vi "Main_Transfer_LaunchPy.vi"() -> ()   [LabVIEW 2020]
uses:
  <vilib>/vision/NI_Vision_Development_Module.lvlib
panel:
  in  "h":i32=10 min=1 max=5000 step=1
  in  "w":i32=1 min=1 max=5000 step=1
  out "Elaps ms":u32
  in  "Send Image":bool
  out "Path to Python script":path
  in  "Stop":bool
  out "Answer":string
  in  "Ping":bool
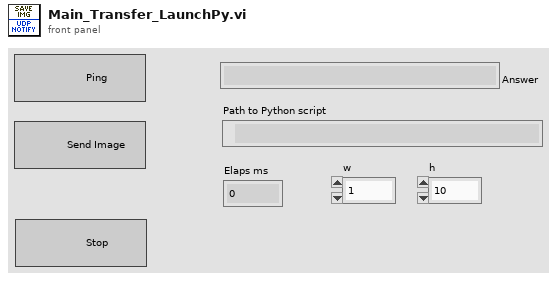
[diagram p1: front panel]
types:
  T1 = enum8{"Enabled", "Disabled", "Disabled and Grayed Out"}
  T2 = typedef "Image Type" = u32
  T3 = cluster{"Rows Per Strip":i32, "Photometric":i32, "Compression Type":i32}
  T4 = typedef "IMAQ Image.ctl" = refnum<image>
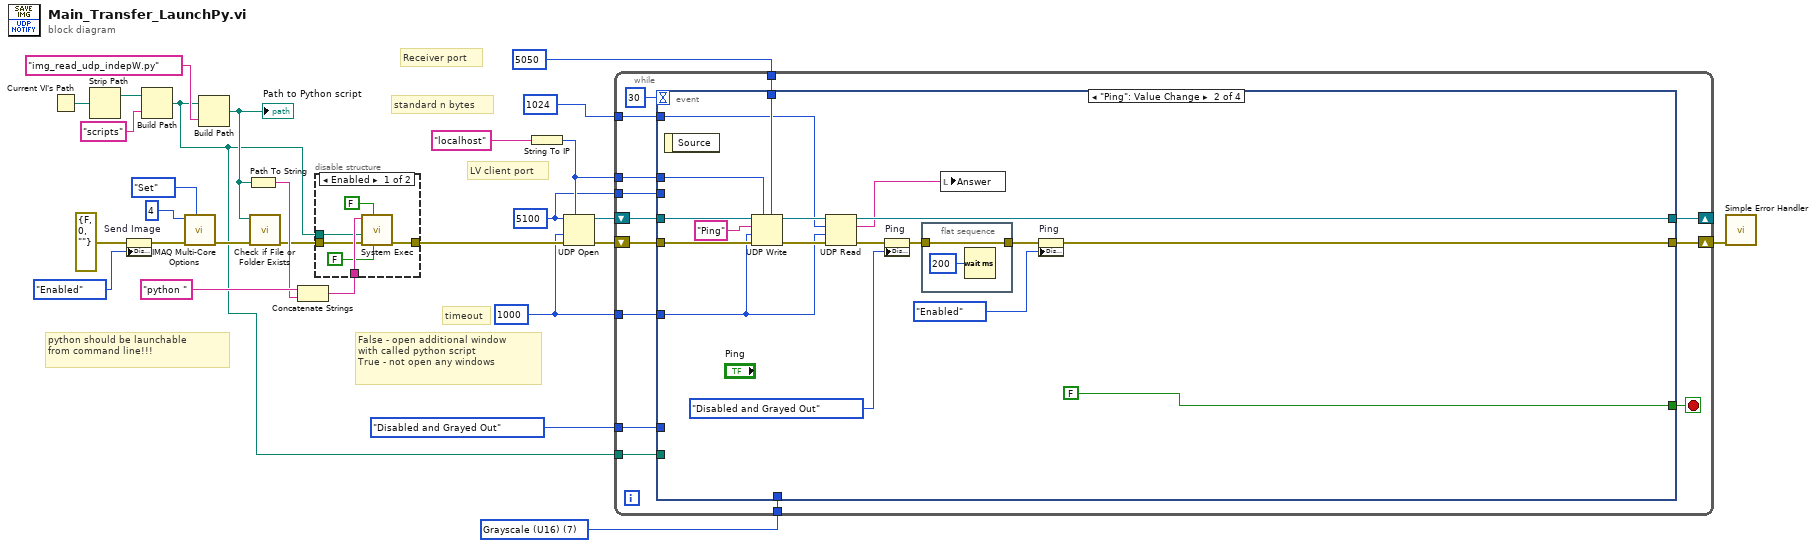
[diagram p0: block diagram]
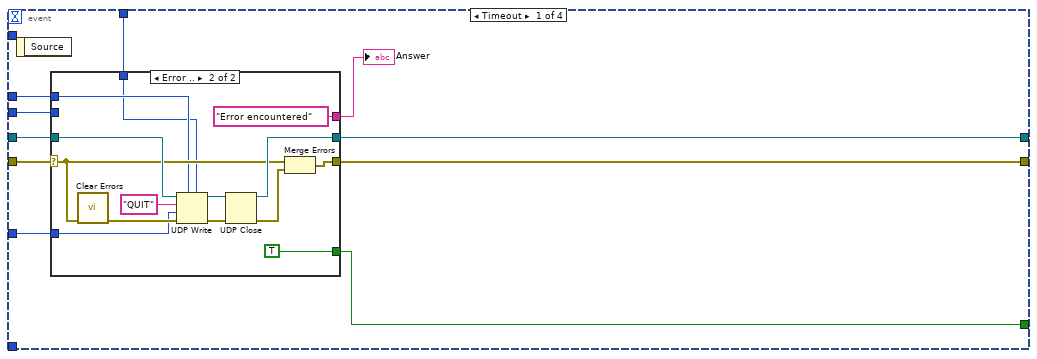
[diagram p3: hidden frame]
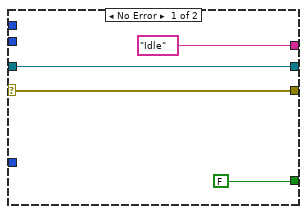
[diagram p4: hidden frame]
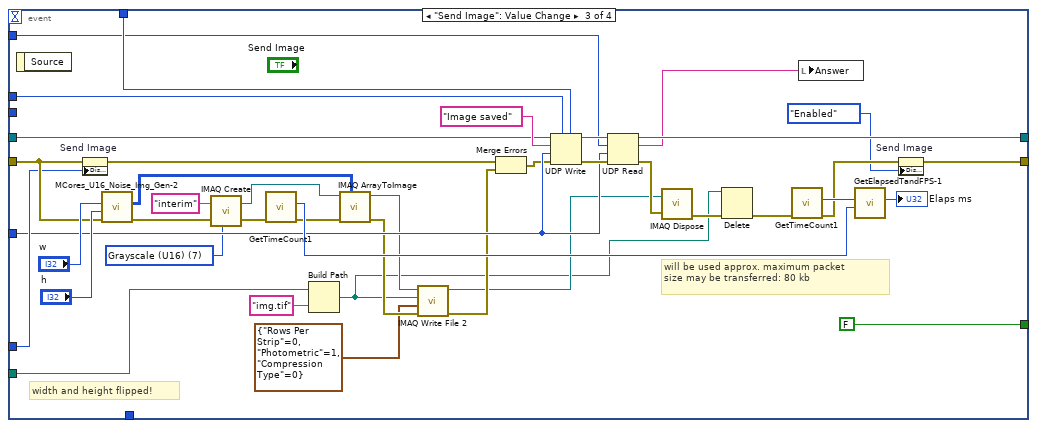
[diagram p5: hidden frame]
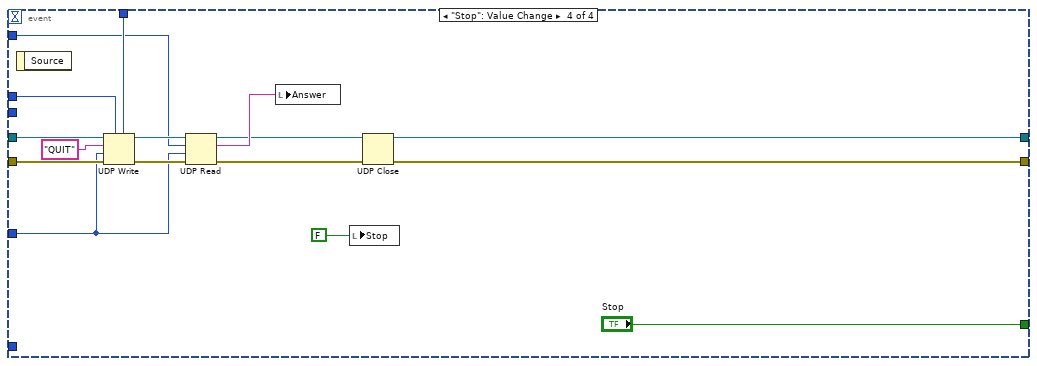
[diagram p6: hidden frame]
diagram:
  w13 = T2 7 items=["Grayscale (U8)", "Grayscale (I16)", "Grayscale (SGL)", "Complex (CSG)", "RGB (U32)", "HSL (U32)", "RGB (U64)", "Grayscale (U16)"] ("Image Type")
  w1 = 1000
  w15 = u16 5100 ("remote port or service name")
  # "standard n bytes"
  # "timeout"
  # "Receiver port"
  # "LV client port"
  # "False - open additional window\nwith called python script\nTrue - not open any windows"
  # "python should be launchable \nfrom command line!!!"
  n1 = Current VI's Path() -> (path=w27:path)
  n2 = Strip Path(path=w27) -> (stripped path=w3:path)  [unwired: 1 out]
  n3 = property on="Send Image" class="Bool"(error in=errorcluster {"status"=FALSE, "code"=0, "source"=""} ("error in (no error)"), "DisabledEnum"=T1."Enabled" ("Disabled")) -> (error out=w7:errorcluster)  [unwired: 1 in, 1 out]
  n4 = Build Path(base path=w3, name or relative path="scripts" ("string")) -> (appended path=w2:path)
  n5 = call "IMAQ Multi-Core Options"("Get/Set Number of Cores (Get)"=enum32{"Get", "Set", "Set Max Available"}."Set", "error in (no error)"=w7, "Specified Number of Cores"=u32 4) -> ("error out"=w4:errorcluster)  [unwired: 7 in, 1 out]
  n6 = Build Path(base path=w2, name or relative path="img_read_udp_indepW.py" ("string")) -> (appended path=w22:path)
  "Path to Python script" <- w22
  n7 = Path To String(path=w22) -> (string=w23:string)
  n8 = call <vilib>:"Check if File or Folder Exists.vi"("error in (no error)"=w4, "path"=w22) -> ("error out"=w21:errorcluster)  [unwired: 7 in, 2 out]
  n9 = Concatenate Strings("python " ("command line"), w23) -> (w25:string)
  n10 = disable-structure shown="Enabled" {
    disable-tunnel: w25 -> [w34 _]
    disable-tunnel: [w33 w35] -> w20
    disable-tunnel: w21 -> [w31 w35]
    disable-tunnel: w2 -> [w29 _]
    frame Enabled {
      n11 = call <vilib>:"System Exec.vi"("run minimized? (F)"=FALSE, "wait until completion? (T)"=FALSE, "error in (no error)"=w31, "working directory"=w29, "command line"=w34) -> ("error out"=w33:errorcluster)  [unwired: 3 in, 3 out]
    }
    frame Disabled {
    }
  }
  n12 = String To IP(1:"localhost" ("address")) -> (0:w16:u32)
  n13 = UDP Open(7:w16, 8:w20, 9:w1, 11:w15) -> (port=w18:refnum<k16>, 0:w19:errorcluster)  [unwired: 1 in, 1 out]
  n14 = while {
    shift-right: [w46] -> _
    shift-left: w18 -> [w47]
    shift-right: [w44] -> w28
    shift-left: w19 -> [w48]
    tunnel: w16 -> [w42]
    tunnel: w15 -> [w43]
    tunnel: u16 5050 ("remote port or service name") -> [w41]
    tunnel: w1 -> [w40]
    tunnel: w13 -> [w39]
    tunnel: T1."Disabled and Grayed Out" ("Disabled") -> [w38]
    tunnel: 1024 ("bytes to read") -> [w37]
    tunnel: w2 -> [w36]
    stop <- w45 stop-if-true
    n15 = event shown="[1] \"Ping\": Value Change" {
      selector: _ -> [_ _ _ _]
      dyn-events: _ -> [_ _ _ _]
      timeout: 30 -> [_ _ _ _]
      tunnel: [w55 FALSE ("Stop") FALSE ("Stop") "Stop"] -> w45
      tunnel: w48 -> [w59 w89 w126 w149]
      tunnel: w47 -> [w58 w88 w137 w150]
      tunnel: [w57 w84 w135 w151] -> w46
      tunnel: [w56 w91 w123 w152] -> w44
      tunnel: w43 -> [w53 _ _ _]
      tunnel: w42 -> [w52 w81 w130 w142]
      tunnel: w41 -> [w51 w80 w129 w141]
      tunnel: w40 -> [w50 w79 w119 w139]
      tunnel: w39 -> [_ _ _ _]
      tunnel: w38 -> [_ _ w125 _]
      tunnel: w37 -> [_ w78 w118 w140]
      tunnel: w36 -> [_ _ w104 _]
      event Timeout {
        n16 = event-data() -> ()  [unwired: 1 in, 1 out]
        n17 = case shown="Error .." w59 {
          selector: w59 -> [w62 w68]
          tunnel: [w63 w75] -> w57
          tunnel: w58 -> [w63 w74]
          tunnel: [w62 w69] -> w56
          tunnel: [FALSE ("Stop") TRUE ("Stop")] -> w55
          tunnel: ["Idle" ("Answer") "Error encountered" ("Answer")] -> w54
          tunnel: w53 -> [_ _]
          tunnel: w52 -> [_ w66]
          tunnel: w51 -> [_ w65]
          tunnel: w50 -> [_ w64]
          frame No Error {
          }
          frame Error {
            n18 = call <vilib>:"Clear Errors.vi"("error in (no error)"=w68) -> ("error out"=w73:errorcluster)  [unwired: 5 in, 1 out]
            n19 = UDP Write(address=w66, port or service name=w65, connection ID=w74, data in="QUIT", 8:w73, 9:w64) -> (error out=w72:errorcluster, 3:w70:refnum<k16>)
            n20 = UDP Close(connection ID=w70, 8:w72) -> (connection ID out=w75:refnum<k16>, error out=w67:errorcluster)
            n21 = Merge Errors(w68, w67) -> (w69:errorcluster)
          }
        }
        "Answer" <- w54
      }
      event "Ping": Value Change {
        n22 = event-data() -> ()  [unwired: 1 in, 1 out]
        n23 = UDP Write(address=w81, port or service name=w80, connection ID=w88, data in="Ping", 8:w89, 9:w79) -> (error out=w86:errorcluster, 3:w85:refnum<k16>)
        n24 = UDP Read(connection ID=w85, max size (548)=w78, timeout ms (25000)=w79, 8:w86) -> (data out=w82:string, error out=w83:errorcluster, 3:w84:refnum<k16>)  [unwired: 2 out]
        n25 = property on="Ping" class="Bool"(error in=w83, "DisabledEnum"=T1."Disabled and Grayed Out" ("Disabled")) -> (error out=w94:errorcluster)  [unwired: 1 in, 1 out]
        n26 = flat-sequence {
          tunnel: w94 -> [w96]
          tunnel: [w96] -> w92
          frame #0 {
            n27 = Wait (ms)(milliseconds to wait=u32 200) -> ()  [unwired: 1 out]
          }
        }
        n28 = local write "Answer"(w82) -> ()
        n29 = property on="Ping" class="Bool"(error in=w92, "DisabledEnum"=T1."Enabled" ("Disabled")) -> (error out=w91:errorcluster)  [unwired: 1 in, 1 out]
      }
      event "Send Image": Value Change {
        w115 = T2 7 items=["Grayscale (U8)", "Grayscale (I16)", "Grayscale (SGL)", "Complex (CSG)", "RGB (U32)", "HSL (U32)", "RGB (U64)", "Grayscale (U16)"] ("Image Type")
        # "width and height flipped!"
        # "will be used approx. maximum packet \nsize may be transferred: 80 kb"
        n30 = event-data() -> ()  [unwired: 1 in, 1 out]
        n31 = property on="Send Image" class="Bool"(error in=w126, "DisabledEnum"=w125) -> (error out=w117:errorcluster)  [unwired: 1 in, 1 out]
        n32 = call "MCores_U16_Noise_Img_Gen-2.vi"("error IN"=w126, "[IN] Width"="h", "[IN] Height"="w") -> ("error OUT"=w113:errorcluster, "[OUT] U16 Pixel Img"=w109:u16[][])  [unwired: 7 in]
        n33 = call "IMAQ Create"("Image Name"="interim", "Image Type"=w115, "error in (no error)"=w113) -> ("New Image"=w110:T4, "error out"=w112:errorcluster)  [unwired: 2 in]
        n34 = call "GetTimeCount1.vi"("error IN"=w112) -> ("error OUT"=w111:errorcluster, "[OUT] Timer Count"=w132:u32)  [unwired: 9 in]
        n35 = Build Path(base path=w104, name or relative path="img.tif" ("string")) -> (appended path=w98:path)
        n36 = call "IMAQ ArrayToImage"("Image Pixels (U16)"=w109, "error in (no error)"=w111, "Image"=w110) -> ("error out"=w108:errorcluster, "Image Out"=w107:T4)  [unwired: 7 in]
        n37 = call-poly "IMAQ Write File 2"("error in (no error)"=w108, "TIFF Options"=T3 {"Rows Per Strip"=0, "Photometric"=1, "Compression Type"=0}, "File Path"=w98, "Image"=w107) -> ("error out"=w106:errorcluster, "Image Out (duplicate)"=w101:T4)  [unwired: 6 in]
        n38 = Merge Errors(w117, w106) -> (w116:errorcluster)
        n39 = UDP Write(address=w130, port or service name=w129, connection ID=w137, data in="Image saved", 8:w116, 9:w119) -> (error out=w120:errorcluster, 3:w121:refnum<k16>)
        n40 = UDP Read(connection ID=w121, max size (548)=w118, timeout ms (25000)=w119, 8:w120) -> (data out=w134:string, error out=w102:errorcluster, 3:w135:refnum<k16>)  [unwired: 2 out]
        n41 = call "IMAQ Dispose"("Image"=w101, "error in (no error)"=w102) -> ("error out"=w100:errorcluster)  [unwired: 4 in]
        n42 = Delete(path (use dialog)=w98, error in=w100) -> (error out=w99:errorcluster)  [unwired: 3 in, 2 out]
        n43 = call "GetTimeCount1.vi"("error IN"=w99) -> ("error OUT"=w124:errorcluster, "[OUT] Timer Count"=w133:u32)  [unwired: 9 in]
        n44 = local write "Answer"(w134) -> ()
        n45 = call "GetElapsedTandFPS-1.vi"("[IN] Timer Count Before ALL [ms]"=w132, "[IN] Timer Count After ALL [ms]"=w133) -> ("[OUT] Elapsed time [ms]"=→"Elaps ms":u32)  [unwired: 3 in, 2 out]
        n46 = property on="Send Image" class="Bool"(error in=w124, "DisabledEnum"=T1."Enabled" ("Disabled")) -> (error out=w123:errorcluster)  [unwired: 1 in, 1 out]
      }
      event "Stop": Value Change {
        n47 = event-data() -> ()  [unwired: 1 in, 1 out]
        n48 = UDP Write(address=w142, port or service name=w141, connection ID=w150, data in="QUIT", 8:w149, 9:w139) -> (error out=w146:errorcluster, 3:w147:refnum<k16>)
        n49 = UDP Read(connection ID=w147, max size (548)=w140, timeout ms (25000)=w139, 8:w146) -> (data out=w144:string, error out=w145:errorcluster, 3:w143:refnum<k16>)  [unwired: 2 out]
        n50 = local write "Answer"(w144) -> ()
        n51 = local write "Stop"(FALSE ("Stop")) -> ()
        n52 = UDP Close(connection ID=w143, 8:w145) -> (connection ID out=w151:refnum<k16>, error out=w152:errorcluster)
      }
    }
  }
  n53 = call <vilib>:"Simple Error Handler.vi"("error in (no error)"=w28) -> ()  [unwired: 4 in, 5 out]
